vi "convert ps to um (speed).vi"(1 "Delay speed (ps/s)":dbl) -> (0 "Position speed (um/s)":dbl)   [LabVIEW 2019, in "Instrument.Aerotech.lvclass"]
uses:
  Instrument.Aerotech.lvclass
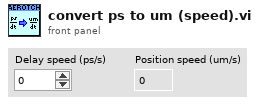
[diagram p1: front panel]
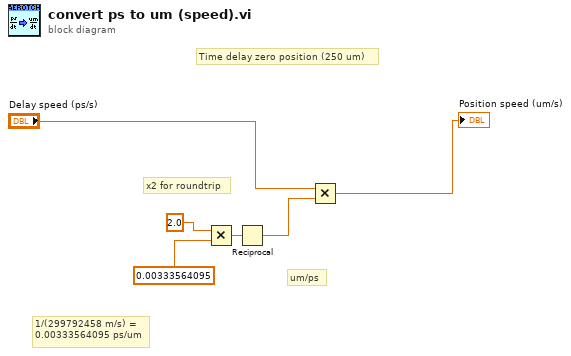
[diagram p0: block diagram]
diagram:
  # "Time delay zero position (250 um)"
  # "um/ps"
  # "1/(299792458 m/s) = \n0.00333564095 ps/um"
  # "x2 for roundtrip"
  n1 = Multiply(x=2.0, y=0.00333564095) -> (x*y=w3:dbl)
  n2 = Reciprocal(x=w3) -> (1/x=w2:dbl)
  n3 = Multiply(x="Delay speed (ps/s)", y=w2) -> (x*y=→"Position speed (um/s)":dbl)
